vi "initialize.vi"() -> ()   [LabVIEW 2020]
panel:
  out "Package Directory":path
  in  "FMC Parameters":T1={"IP"="169.254.92.202", "Port"=22, "Username"="analog", "Password"="analog"}
  out "Error Out":errorcluster
  out "Terminal Output":string
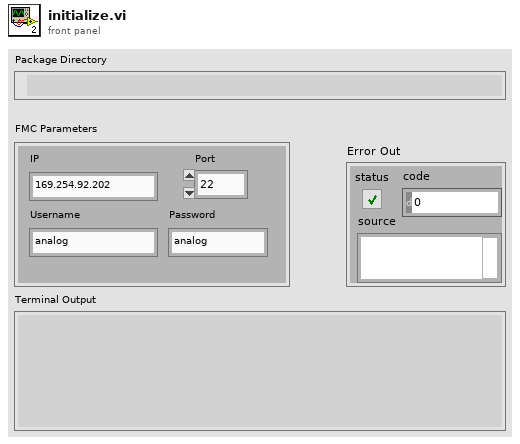
[diagram p1: front panel]
types:
  T1 = cluster{"IP":string, "Port":i32, "Username":string, "Password":string}
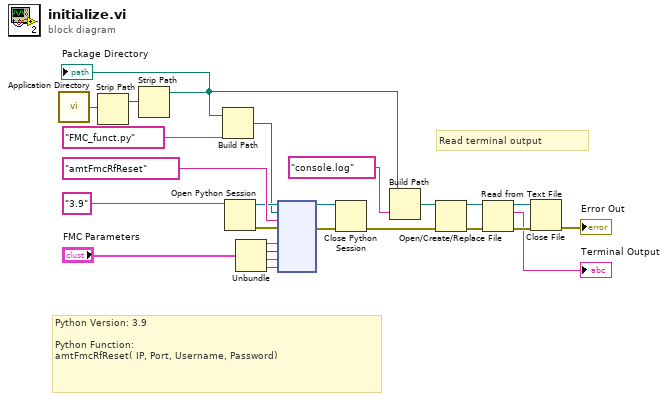
[diagram p0: block diagram]
diagram:
  # "Read terminal output"
  # "Python Version: 3.9\n\nPython Function:\namtFmcRfReset( IP, Port, Username, Password)"
  n1 = call <vilib>:"Application Directory.vi"() -> ("Application Directory"=w2:path)
  n2 = Strip Path(path=w2) -> (stripped path=w3:path)  [unwired: 1 out]
  n3 = Strip Path(path=w3) -> (stripped path=w1:path)  [unwired: 1 out]
  "Package Directory" <- w1
  n4 = Build Path(base path=w1, name or relative path="FMC_funct.py") -> (appended path=w15:path)
  n5 = Open Python Session(python version="3.9" ("Python version")) -> (session out=w23:refnum<k35>, error out=w22:errorcluster)  [unwired: 2 in]
  n6 = Unbundle("FMC Parameters") -> ("IP"=w18:string, "Port"=w19:i32, "Username"=w20:string, "Password"=w21:string)
  n7 = node(w23, w15, "amtFmcRfReset" ("function name"), w22, w18, w19, w20, w21) -> (w14:refnum<k35>, w13:errorcluster)  [unwired: 6 in, 2 out]
  n8 = Close Python Session(session in=w14, error in=w13) -> (11:w6:errorcluster)
  n9 = Build Path(base path=w1, name or relative path="console.log" ("function name")) -> (appended path=w7:path)
  n10 = Open/Create/Replace File(file path (use dialog)=w7, error in=w6) -> (refnum out=w12:refnum<file>, error out=w9:errorcluster)  [unwired: 4 in, 1 out]
  n11 = Read from Text File(file (use dialog)=w12, error in=w9) -> (refnum out=w11:refnum<file>, text=→"Terminal Output":string, error out=w10:errorcluster)  [unwired: 2 in, 1 out]
  n12 = Close File(refnum=w11, error in=w10) -> (error out=→"Error Out":errorcluster)  [unwired: 1 out]
